vi "GPIB_Write&Read.vi"(7 "Read?":bool=TRUE, 8 "error in (no error)":errorcluster, 9 "String":string, 10 "wait ms":i32=100, 11 "GPIB Addr":string) -> (0 "error out":errorcluster, 2 "read buffer":string)   [LabVIEW 2013]
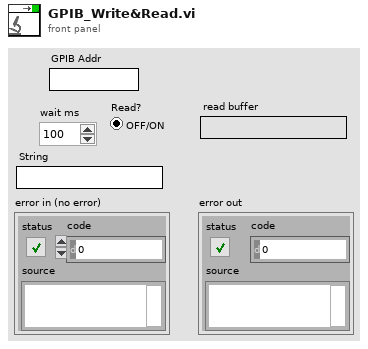
[diagram p1: front panel]
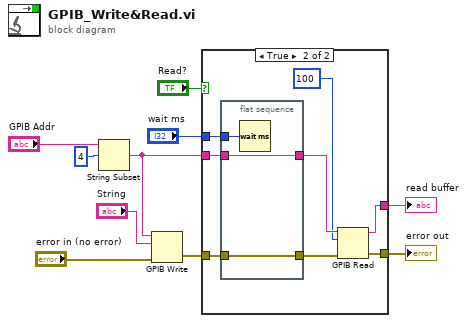
[diagram p0: block diagram]
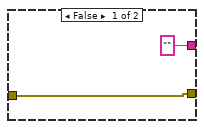
[diagram p2: hidden frame]
diagram:
  n1 = String Subset(string="GPIB Addr", offset (0)=4) -> (substring=w1:string)  [unwired: 1 in]
  n2 = GPIB Write(0:w1, 1:"String", 3:"error in (no error)") -> (6:w4:errorcluster)  [unwired: 2 in, 1 out]
  n3 = case shown="True" "Read?" {
    tunnel: ["" ("read buffer") w18] -> w10
    tunnel: [w12 w14] -> w9
    tunnel: "wait ms" -> [_ w20]
    tunnel: w4 -> [w12 w19]
    tunnel: w1 -> [_ w17]
    frame False {
    }
    frame True {
      n4 = flat-sequence {
        tunnel: w20 -> [w23]
        tunnel: [w22] -> w15
        tunnel: w19 -> [w22]
        tunnel: w17 -> [w21]
        tunnel: [w21] -> w16
        frame #0 {
          n5 = Wait (ms)(milliseconds to wait=w23) -> ()  [unwired: 1 out]
        }
      }
      n6 = GPIB Read(0:w16, 1:100 ("byte count"), 3:w15) -> (5:w18:string, 7:w14:errorcluster)  [unwired: 2 in, 1 out]
    }
  }
  "read buffer" <- w10
  "error out" <- w9
